vi "计算低频Z.vi"(0 "特性阻抗Z0":dbl, 7 "factor":dbl, 9 "L":dbl, 11 "H43":cdb[](array[numeric]), 12 "k":cdb[](array[numeric])) -> (4 "Z低频":cdb[](array[numeric]))   [LabVIEW 2018]
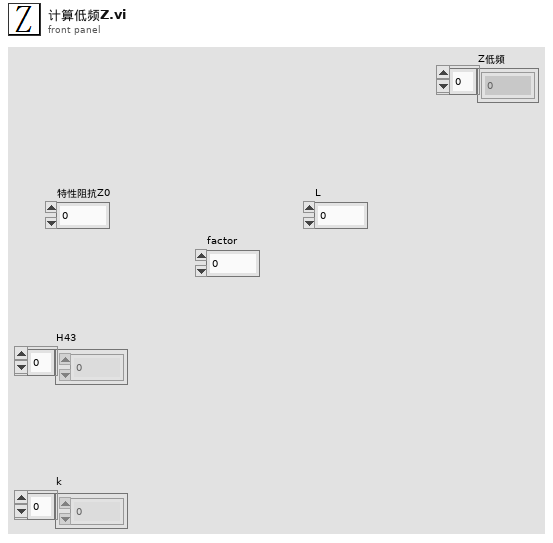
[diagram p1: front panel]
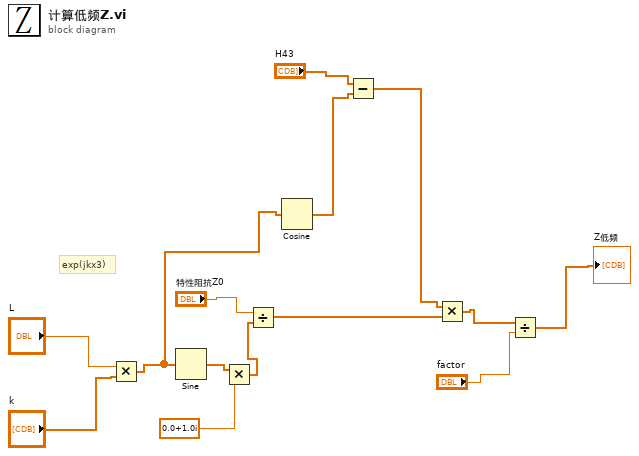
[diagram p0: block diagram]
diagram:
  # "exp(jkx3)"
  n1 = Multiply(x="L", y="k") -> (x*y=w6:cdb[])
  n2 = Sine(x=w6) -> (sin(x)=w12:cdb[])
  n3 = Multiply(x=w12, y=cdb 0.0+1.0i) -> (x*y=w10:cdb[])
  n4 = Divide(x="特性阻抗Z0", y=w10) -> (x/y=w9:cdb[])
  n5 = Cosine(x=w6) -> (cos(x)=w5:cdb[])
  n6 = Subtract(x="H43", y=w5) -> (x-y=w8:cdb[])
  n7 = Multiply(x=w8, y=w9) -> (x*y=w4:cdb[])
  n8 = Divide(x=w4, y="factor") -> (x/y=→"Z低频":cdb[])
